vi "Telnet_Cmd.vi"(8 "Error In":errorcluster caption="Entrée d'erreur", 9 "Cmd":string, 10 "Timeout (ms)":u32=1000, 11 "Host":cluster{"IP":string, "Port":u16}={"IP"="0.0.0.0", "Port"=0}) -> (0 "Error Out":errorcluster caption="Sortie d'erreur", 2 "DataLines":string[](array[string]), 3 "DataString":string, 5 "Console":string)   [LabVIEW 2013]
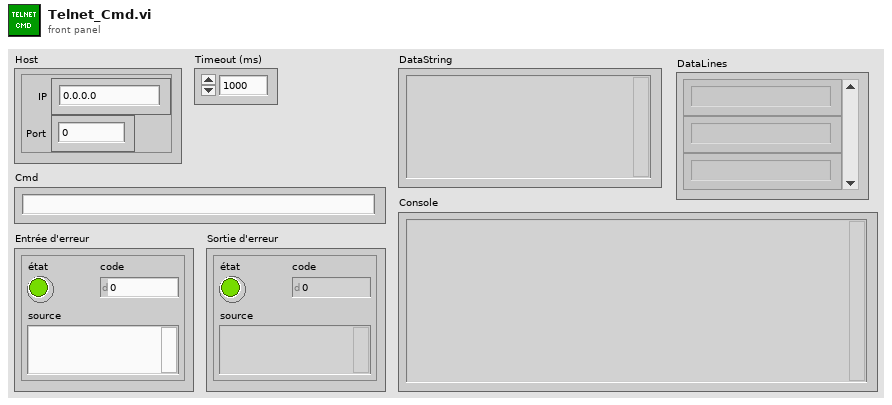
[diagram p1: front panel]
types:
  T1 = typedef "Telnet Session.ctl" = refnum<k1>
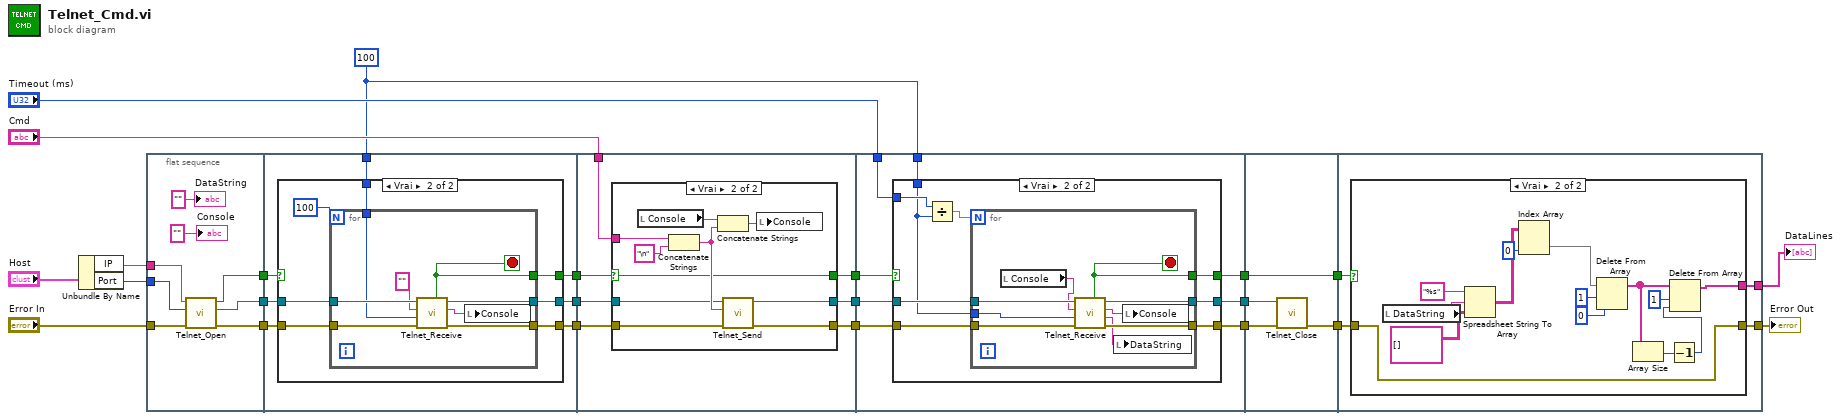
[diagram p0: block diagram]
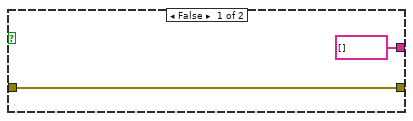
[diagram p5: hidden frame]
diagram:
  w9 = u32 100 ("attente (ms)")
  n1 = Unbundle By Name("Host") -> ("IP"=w6:string, "Port"=w5:u16)
  n2 = flat-sequence {
    tunnel: w6 -> [w31]
    tunnel: "Error In" -> [w30]
    tunnel: [w29] -> w22
    tunnel: [w28] -> w21
    tunnel: [w27] -> w20
    tunnel: w5 -> [w24]
    tunnel: [w35] -> w19
    tunnel: [w34] -> w18
    tunnel: [w33] -> w11
    tunnel: w20 -> [w36]
    tunnel: w21 -> [w37]
    tunnel: w22 -> [w38]
    tunnel: w9 -> [w32]
    tunnel: w19 -> [w61]
    tunnel: w18 -> [w62]
    tunnel: "Cmd" -> [w63]
    tunnel: [w59] -> w16
    tunnel: [w60] -> w15
    tunnel: w11 -> [w58]
    tunnel: [w57] -> w10
    tunnel: w16 -> [w81]
    tunnel: w15 -> [w82]
    tunnel: "Timeout (ms)" -> [w80]
    tunnel: [w84] -> w13
    tunnel: w10 -> [w83]
    tunnel: w9 -> [w79]
    tunnel: [w78] -> w8
    tunnel: [w77] -> w2
    tunnel: w13 -> [w108]
    tunnel: w8 -> [w106]
    tunnel: [w107] -> w4
    tunnel: [w105] -> w3
    tunnel: w2 -> [w105]
    tunnel: [w112] -> w12
    tunnel: w4 -> [w111]
    tunnel: w3 -> [w110]
    tunnel: [w109] -> w1
    frame #0 {
      n3 = call "Telnet_Open.vi"("Error In"=w30, "RemotePort(23)"=w24, "HostAddress"=w31) -> ("Error Out"=w29:errorcluster, "telnet connection"=w28:T1, "Status"=w27:bool)  [unwired: 6 in]
      "Console" <- "" ("Console in")
      "DataString" <- "" ("DataIn")
    }
    frame #1 {
      n4 = case shown="Vrai" w36 {
        selector: w36 -> [w40 _]
        tunnel: w38 -> [w41 w48]
        tunnel: w37 -> [w39 w47]
        tunnel: [w41 w44] -> w35
        tunnel: [w40 w46] -> w33
        tunnel: [w39 w45] -> w34
        tunnel: w32 -> [_ w42]
        frame False {
        }
        frame True {
          n5 = for {
            N: u32 100 ("attente (ms)") -> [_]
            tunnel: w48 -> [w56]
            tunnel: w47 -> [w55]
            tunnel: [w50] -> w46
            tunnel: [w53] -> w45
            tunnel: [w52] -> w44
            tunnel: w42 -> [w49]
            stop <- w50 stop-if-true
            n6 = call "Telnet_Receive.vi"("Error In"=w56, "timeout ms (100)"=w49, "Console in"="", "telnet connection in"=w55) -> ("Error Out"=w52:errorcluster, "Console out"=w51:string, "telnet connection out"=w53:T1, "NewData"=w50:bool)  [unwired: 3 in, 1 out]
            n7 = local write "Console"(w51) -> ()
          }
        }
      }
    }
    frame #2 {
      n8 = case shown="Vrai" w58 {
        selector: w58 -> [w64 w67]
        tunnel: w63 -> [_ w72]
        tunnel: w62 -> [w65 w71]
        tunnel: w61 -> [w66 w70]
        tunnel: [w65 w69] -> w60
        tunnel: [w66 w68] -> w59
        tunnel: [w64 w67] -> w57
        frame False {
        }
        frame True {
          n9 = local read "Console"() -> (w76:string)
          n10 = Concatenate Strings(w72, "\n") -> (w73:string)
          n11 = Concatenate Strings(w76, w73) -> (w75:string)
          n12 = call "Telnet_Send.vi"("Error In"=w70, "Data in"=w73, "telnet connection in"=w71) -> ("Error Out"=w68:errorcluster, "telnet connection out"=w69:T1)  [unwired: 7 in]
          n13 = local write "Console"(w75) -> ()
        }
      }
    }
    frame #3 {
      n14 = case shown="Vrai" w83 {
        selector: w83 -> [w86 _]
        tunnel: w81 -> [w87 w95]
        tunnel: w82 -> [w85 w94]
        tunnel: [w87 w91] -> w84
        tunnel: [w86 w93] -> w77
        tunnel: [w85 w92] -> w78
        tunnel: w80 -> [_ w90]
        tunnel: w79 -> [_ w89]
        frame False {
        }
        frame True {
          n15 = Divide(x=w90, y=w89) -> (x/y=w88:dbl)
          n16 = for {
            N: w88 -> [_]
            tunnel: w95 -> [w104]
            tunnel: w94 -> [w103]
            tunnel: [w99] -> w93
            tunnel: [w102] -> w92
            tunnel: [w101] -> w91
            tunnel: w89 -> [w96]
            stop <- w99 stop-if-true
            n17 = local read "Console"() -> (w98:string)
            n18 = call "Telnet_Receive.vi"("Error In"=w104, "timeout ms (100)"=w96, "Console in"=w98, "telnet connection in"=w103) -> ("Error Out"=w101:errorcluster, 1:"NewData"=w97:string, "Console out"=w100:string, "telnet connection out"=w102:T1, 5:"NewData"=w99:bool)  [unwired: 3 in]
            n19 = local write "DataString"(w97) -> ()
            n20 = local write "Console"(w100) -> ()
          }
        }
      }
    }
    frame #4 {
      n21 = call "Telnet_Close.vi"("Error In"=w108, "telnet connection"=w106) -> ("Error Out"=w107:errorcluster)  [unwired: 8 in, 1 out]
    }
    frame #5 {
      n22 = case shown="Vrai" w110 {
        tunnel: [w114 w125] -> w112
        tunnel: w111 -> [w114 w125]
        tunnel: [string[] [] w115] -> w109
        frame False {
        }
        frame True {
          n23 = local read "DataString"() -> (w127:string)
          n24 = Spreadsheet String To Array(format string="%s" ("chaîne de type tableur"), spreadsheet string=w127, array type (2D Dbl)=string[][] []) -> (array=w124:string[][])  [unwired: 1 in]
          n25 = Index Array(array=w124, index (col)=0 ("indice désactivé (col)")) -> (element=w122:string[])  [unwired: 1 in]
          n26 = Delete From Array(array=w122, length=1 ("longueur"), index=0 ("indice")) -> (array with subset deleted=w118:string[])  [unwired: 1 out]
          n27 = Array Size(array=w118) -> (size(s)=w117:i32)
          n28 = Decrement(x=w117) -> (x-1=w116:i32)
          n29 = Delete From Array(array=w118, length=1 ("longueur"), index=w116) -> (array with subset deleted=w115:string[])  [unwired: 1 out]
        }
      }
    }
  }
  "Error Out" <- w12
  "DataLines" <- w1
